vi "Create Sysdef and Add New Custom Device from Spreadsheet.vi"() -> ()   [LabVIEW 2010]
uses:
  NationalInstruments.VeriStand.SystemDefinitionAPI
  Read RefMem PtByPt System Definition API.lvlibp
panel:
  out "Range Warning":bool
  in  "SpreadSheet To Load":path
  in  "Decimation":i32=1
  in  "VISA Name":string="RM"
  in  "Device Name":string="My RefMem"
  in  "Sysdef File to create":path
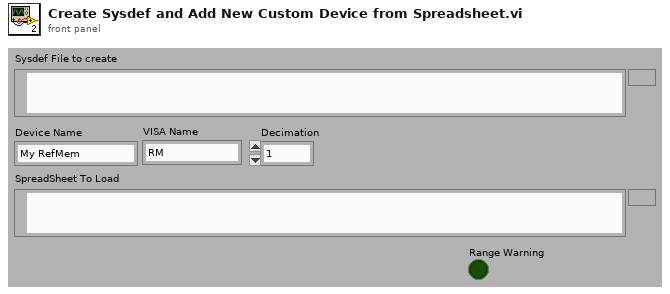
[diagram p1: front panel]
types:
  T1 = typedef "SysDefRefs.ctl" = cluster{"SysDef Ref":refnum<k24>, "Root Node":refnum<k24>, "Targets Section":refnum<k24>, "Target List":refnum<k24>[], "CD Section":refnum<k24>, "CustomDeviceList":refnum<k24>[]}
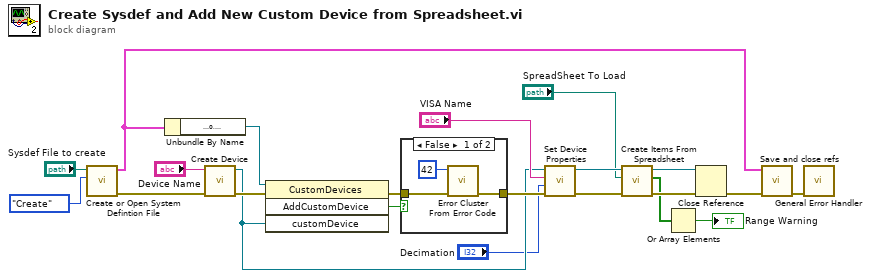
[diagram p0: block diagram]
diagram:
  n1 = call "Create or Open System Defintion File.vi"("File Action"=enum16{"Open", "Create"}."Create", "Sysdef File"="Sysdef File to create") -> ("error out"=w14:errorcluster, "SysDef Refs"=w18:T1)  [unwired: 8 in]
  n2 = Unbundle By Name(w18) -> ("CD Section"=w17:refnum<k24>)
  n3 = call "Create Device.vi"("error in (no error)"=w14, "Name"="Device Name") -> ("error out"=w11:errorcluster, "Custom Device"=w9:refnum<k24>)  [unwired: 8 in]
  n4 = invoke class="CustomDevices" method="AddCustomDevice"(reference=w17, error in=w11, "customDevice"=w9) -> (error out=w20:errorcluster, "AddCustomDevice"=w19:bool)  [unwired: 1 in, 2 out]
  n5 = case shown="False" w19 {
    tunnel: [w24 w26] -> w10
    tunnel: w20 -> [w23 w26]
    frame False {
      n6 = call <vilib>:"Error Cluster From Error Code.vi"("error in (no error)"=w23, "error code (0)"=42) -> ("error out"=w24:errorcluster)  [unwired: 7 in]
    }
    frame True {
    }
  }
  n7 = call "Set Device Properties.vi"("error in (no error)"=w10, "Decimation"="Decimation", "VISA Name"="VISA Name", "Custom Device"=w9) -> ("error out"=w7:errorcluster, "Custom Device Duplicate"=w6:refnum<k24>)  [unwired: 6 in]
  n8 = call "Create Items From Spreadsheet.vi"("error in (no error)"=w7, "file path (use dialog)"="SpreadSheet To Load", "Custom Device"=w6) -> ("error out"=w5:errorcluster, "Channel Created Inside NIVS Address Range"=w2:bool[], "Custom Device Duplicate"=w4:refnum<k24>)  [unwired: 6 in]
  n9 = Or Array Elements(Boolean array=w2) -> (logical OR=→"Range Warning":bool)
  n10 = Close Reference(reference=w4, error in (no error)=w5) -> (error out=w12:errorcluster)
  n11 = call "Save and close refs.vi"("error in (no error)"=w12, "SysDef Refs in"=w18) -> ("error out"=w21:errorcluster)  [unwired: 9 in]
  n12 = call <vilib>:"General Error Handler.vi"("error in (no error)"=w21) -> ()  [unwired: 10 in, 5 out]
